vi "LVClass_Pupil Barycentre.vi"(0 "Pupil in":refnum<class "Pupil.lvclass">, 11 "error in (no error)":errorcluster) -> (4 "Pupil out":refnum<class "Pupil.lvclass">, 8 "barycentre_um":T1, 15 "error out":errorcluster)   [LabVIEW 2020, in "Pupil.lvclass"]
doc: "Get Pupil barycenter.\n\n--------------------------------------------------------------------------------\n\n<B>PupilIn </B> : Pupil object.\n<B>PupilOut </B> : Pupil object.\n<B>barycenter </B> : Pupil barycenter.\n<B>ErrorIn </B> : Error\n<B>ErrorOut </B> : Error\n\n--------------------------------------------------------------------------------"
uses:
  Pupil.lvclass
  Controls/Point2Df.ctl
  Pupil.lvclass/Pupil.ctl
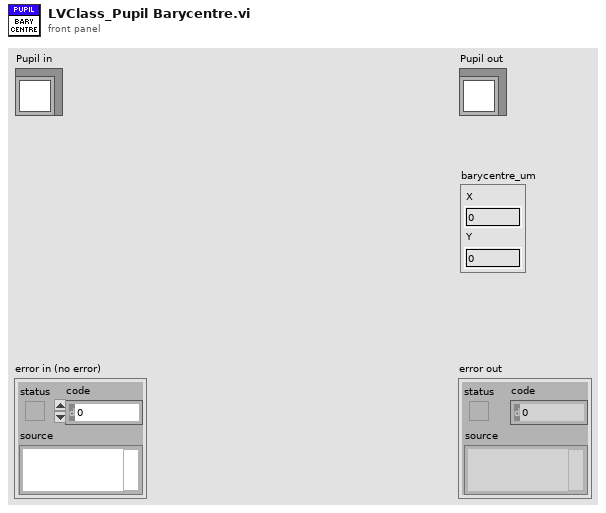
[diagram p1: front panel]
types:
  T1 = typedef "Point2Df.ctl" = cluster{"X":sgl, "Y":sgl}
  T2 = typedef "ClassID.ctl" = i64
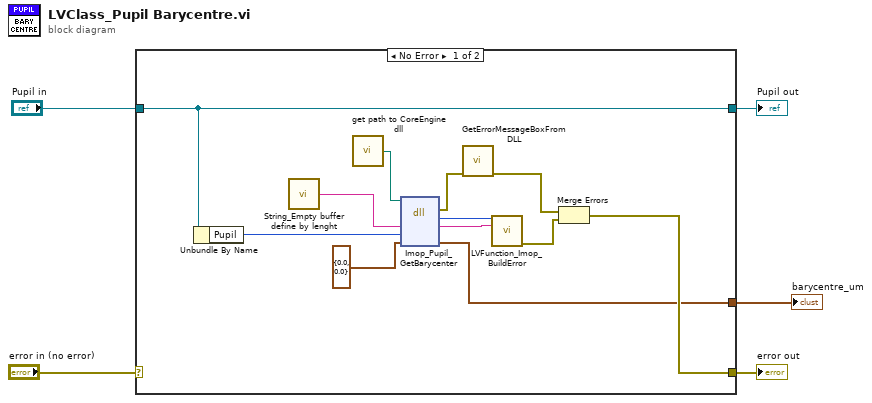
[diagram p0: block diagram]
diagram:
  n1 = case shown="No Error" "error in (no error)" {
    selector: "error in (no error)" -> [_ w19]
    tunnel: [w7 w19] -> w5
    tunnel: [w12 w18] -> w4
    tunnel: "Pupil in" -> [w12 w18]
    tunnel: [w6 _] -> w3
    frame No Error {
      n2 = Unbundle By Name(w12) -> ("Pupil"=w11:T2)
      n3 = call "String_Empty buffer define by lenght.vi"() -> ("Empty buffer"=w17:string)  [unwired: 1 in]
      n4 = call "get path to CoreEngine dll.vi"() -> ("path to wavekit library"=w14:path)  [unwired: 14 in, 1 out]
      n5 = dll-call lib="D:/soft/HASO_v3/SVN_trunk/ImOpCoreEngine4_LV2011/DLLs/c_interface_vc100.dll" fn="Imop_Pupil_GetBarycenter"(path in=w14, "message"=w17, "objet"=w11, "barycentre"=T1 {"X"=0.0, "Y"=0.0} ("Step")) -> (error out=w13:errorcluster, "return type"=w15:i32, "message"=w16:string, "barycentre"=w6:T1)  [unwired: 3 in, 1 out]
      n6 = call "GetErrorMessageBoxFromDLL.vi"("error IN"=w13) -> ("error OUT"=w9:errorcluster)  [unwired: 10 in]
      n7 = call "LVFunction_Imop_BuildError.vi"("code"=w15, "String to Prepend to source (\"\")"=w16) -> ("error out"=w8:errorcluster)  [unwired: 13 in]
      n8 = Merge Errors(w9, w8) -> (w7:errorcluster)
    }
    frame Error {
    }
  }
  "error out" <- w5
  "Pupil out" <- w4
  "barycentre_um" <- w3
